vi "EnergyStorage_Read Status.vi"(11 "EnergyStorage in":refnum<class "EnergyStorage.lvclass">) -> (2 "EnergyStorage_Status":T1, 3 "EnergyStorage out":refnum<class "EnergyStorage.lvclass">)   [LabVIEW 2015, in "EnergyStorage.lvclass"]
uses:
  EnergyStorage.lvclass
  EnergyStorage_Status.ctl
  EnergyStorage.lvclass/EnergyStorage.ctl
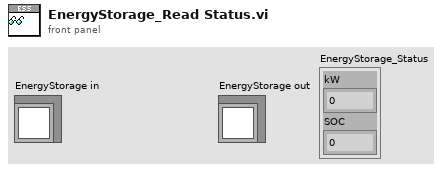
[diagram p1: front panel]
types:
  T1 = typedef "EnergyStorage.lvclass/EnergyStorage_Status.ctl" = cluster{"kW":dbl, "SOC":dbl}
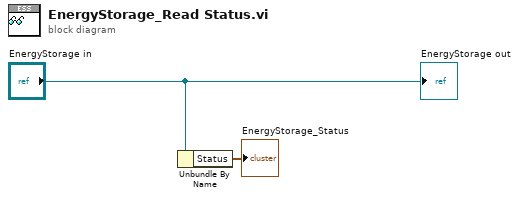
[diagram p0: block diagram]
diagram:
  n1 = Unbundle By Name("EnergyStorage in") -> ("Status"=→"EnergyStorage_Status":T1)
  "EnergyStorage out" <- "EnergyStorage in"
